vi "ImageLoader.vi"(0 "Filename":path, 1 "Load Image":bool) -> (3 "Frame 1":sgl[][](graph))   [LabVIEW 2014]
uses:
  ATSIFIO64.llb/ATSIF_ReadMode Enum.ctl
  ATSIFIO64.llb/ATSIF_DataSource Enum.ctl
panel:
  in  "stop":bool
  out "Sub Image Size":u32
  out "Sub Image Height":u32
  out "Sub Image Width":u32
  out "Image Data":sgl[](array[numeric])
  out "SubImageInfo":T1
  out "Frame Size":u32
  out "Number ofSub Images":u32
  out "Number of Frames":u32
  out "Source Present":i32
  in  "ATSIF_DataSource":T2
  out "Loaded":i32
  in  "ATSIF_ReadMode":T3
  in  "SIFPropertyValue":string
  out "SIF Property - Formatted Time":string
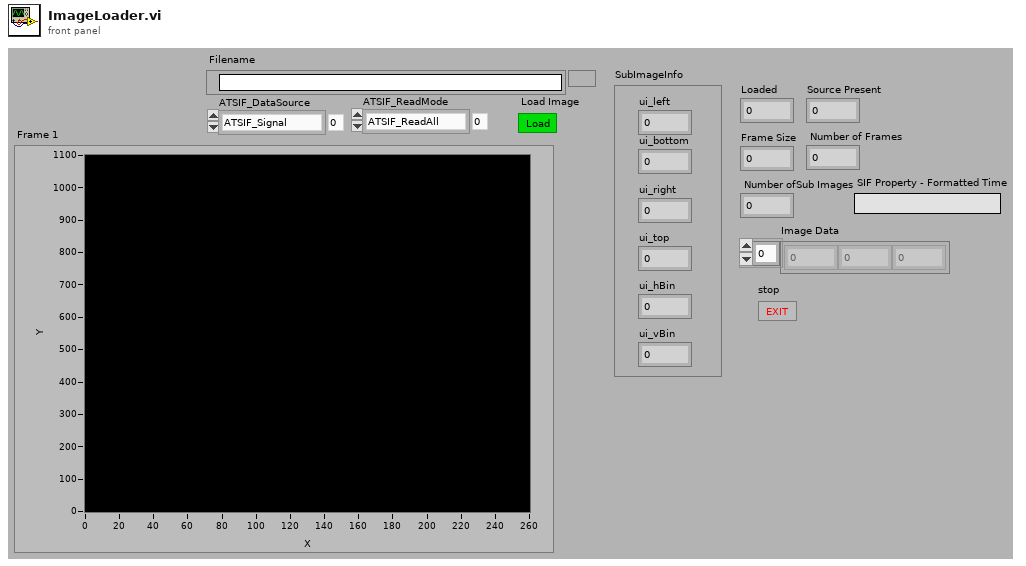
[diagram p1: front panel]
types:
  T1 = cluster{"ui_left":u32, "ui_bottom":u32, "ui_right":u32, "ui_top":u32, "ui_hBin":u32, "ui_vBin":u32}
  T2 = typedef "ATSIF_DataSource Enum.ctl" = enum16{"ATSIF_Signal", "ATSIF_Reference", "ATSIF_Background", "ATSIF_Live", "ATSIF_Source"}
  T3 = typedef "ATSIF_ReadMode Enum.ctl" = enum16{"ATSIF_ReadAll", "ATSIF_ReadHeaderOnly"}
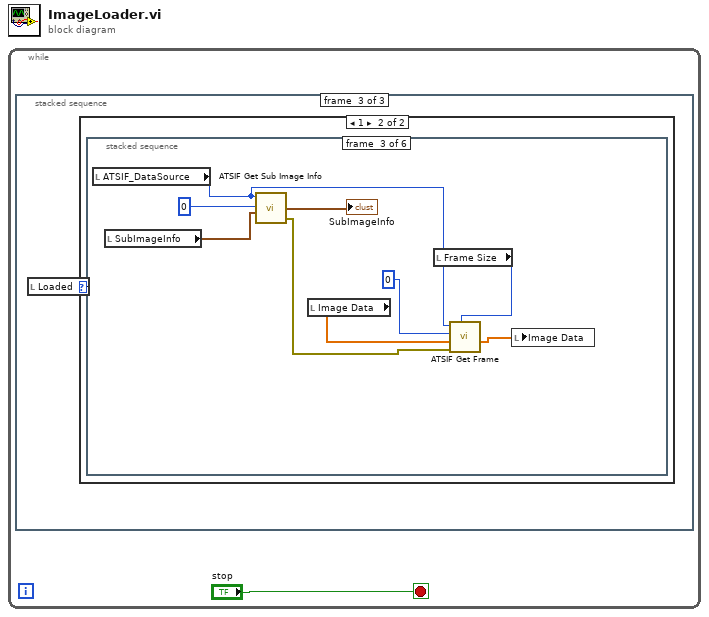
[diagram p0: block diagram]
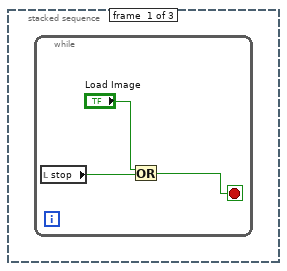
[diagram p2: hidden frame]
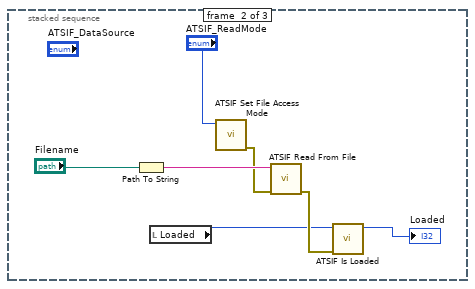
[diagram p3: hidden frame]
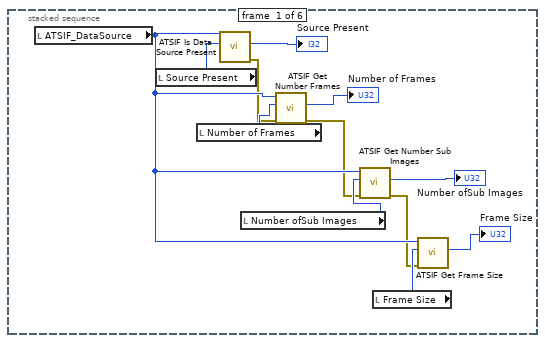
[diagram p5: hidden frame]
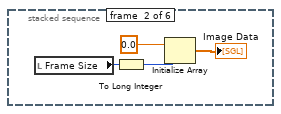
[diagram p6: hidden frame]
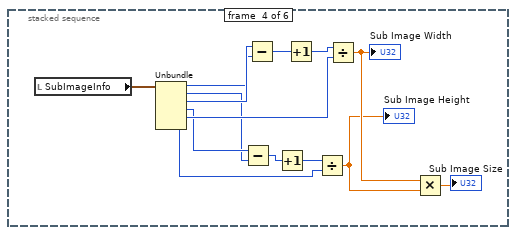
[diagram p7: hidden frame]
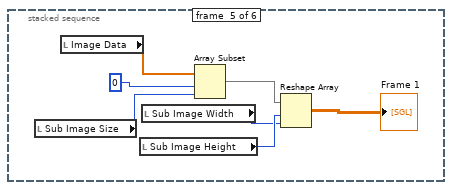
[diagram p8: hidden frame]
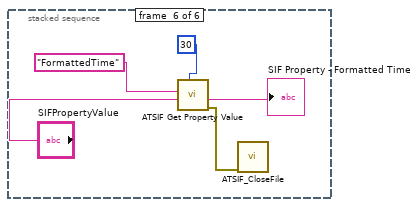
[diagram p9: hidden frame]
diagram:
  n1 = while {
    stop <- "stop" stop-if-true
    n2 = stacked-sequence {
      frame #0 {
        n3 = while {
          stop <- w3 stop-if-true
          n4 = local read "stop"() -> (w2:bool)
          n5 = Or(x="Load Image", y=w2) -> (x .or. y?=w3:bool)
        }
      }
      frame #1 {
        n6 = Path To String(path="Filename") -> (string=w11:string)
        n7 = local read "Loaded"() -> (w5:i32)
        n8 = call "ATSIF Set File Access Mode.vi"("_mode"="ATSIF_ReadMode") -> ("error out"=w7:errorcluster)  [unwired: 1 in, 9 out]
        n9 = call "ATSIF Read From File.vi"("error in (no error)"=w7, "_sz_filename"=w11) -> ("error out"=w9:errorcluster)  [unwired: 9 out]
        n10 = call "ATSIF Is Loaded.vi"("error in (no error)"=w9, "_i_loaded"=w5) -> ("_i_loaded out"=→"Loaded":i32)  [unwired: 9 out]
      }
      frame #2 {
        n11 = local read "Loaded"() -> (w12:i32)
        n12 = case shown="1" w12 {
          frame 0, Default {
          }
          frame 1 {
            n13 = stacked-sequence {
              frame #0 {
                n14 = local read "ATSIF_DataSource"() -> (w21:T2)
                n15 = local read "Source Present"() -> (w20:i32)
                n16 = local read "Number of Frames"() -> (w22:u32)
                n17 = call "ATSIF Is Data Source Present.vi"("_i_present"=w20, "_source"=w21) -> ("error out"=w18:errorcluster, "_i_present out"=→"Source Present":i32)  [unwired: 1 in, 7 out]
                n18 = local read "Number ofSub Images"() -> (w23:u32)
                n19 = call "ATSIF Get Number Frames.vi"("error in (no error)"=w18, "_ui_images"=w22, "_source"=w21) -> ("error out"=w16:errorcluster, "_ui_images out"=→"Number of Frames":u32)  [unwired: 7 out]
                n20 = call "ATSIF Get Number Sub Images.vi"("error in (no error)"=w16, "_ui_subimages"=w23, "_source"=w21) -> ("error out"=w14:errorcluster, "_ui_subimages out"=→"Number ofSub Images":u32)  [unwired: 7 out]
                n21 = local read "Frame Size"() -> (w24:u32)
                n22 = call "ATSIF Get Frame Size.vi"("error in (no error)"=w14, "_ui_size"=w24, "_source"=w21) -> ("_ui_size out"=→"Frame Size":u32)  [unwired: 8 out]
              }
              frame #1 {
                n23 = local read "Frame Size"() -> (w27:u32)
                n24 = To Long Integer(number=w27) -> (32bit integer=w26:i32)
                n25 = Initialize Array(sgl 0.0, w26) -> (→"Image Data":sgl[])
              }
              frame #2 {
                n26 = local read "ATSIF_DataSource"() -> (w32:T2)
                n27 = local read "SubImageInfo"() -> (w35:T1)
                n28 = call "ATSIF Get Sub Image Info.vi"("SubImageInfo"=w35, "_ui_index"=0, "_source"=w32) -> ("error out"=w33:errorcluster, "SubImageInfo out"=→"SubImageInfo":T1)  [unwired: 1 in, 1 out]
                n29 = local read "Image Data"() -> (w29:sgl[])
                n30 = local read "Frame Size"() -> (w31:u32)
                n31 = call "ATSIF Get Frame.vi"("_ui_bufferSize"=w31, "error in (no error)"=w33, "_pf_data"=w29, "_ui_index"=u32 0, "_source"=w32) -> ("_pf_data out"=w30:sgl[])  [unwired: 6 out]
                n32 = local write "Image Data"(w30) -> ()
              }
              frame #3 {
                n33 = local read "SubImageInfo"() -> (w51:T1)
                n34 = Unbundle(w51) -> ("ui_left"=w49:u32, "ui_bottom"=w44:u32, "ui_right"=w50:u32, "ui_top"=w45:u32, "ui_hBin"=w46:u32, "ui_vBin"=w41:u32)
                n35 = Subtract(x=w45, y=w44) -> (x-y=w43:u32)
                n36 = Subtract(x=w50, y=w49) -> (x-y=w48:u32)
                n37 = Increment(x=w43) -> (x+1=w42:u32)
                n38 = Increment(x=w48) -> (x+1=w47:u32)
                n39 = Divide(x=w42, y=w41) -> (x/y=w38:dbl)
                "Sub Image Height" <- w38
                n40 = Divide(x=w47, y=w46) -> (x/y=w39:dbl)
                "Sub Image Width" <- w39
                n41 = Multiply(x=w39, y=w38) -> (x*y=→"Sub Image Size":dbl)
              }
              frame #4 {
                n42 = local read "Sub Image Size"() -> (w56:u32)
                n43 = local read "Image Data"() -> (w58:sgl[])
                n44 = local read "Sub Image Height"() -> (w54:u32)
                n45 = local read "Sub Image Width"() -> (w53:u32)
                n46 = Array Subset(array=w58, index=0, length=w56) -> (w55:sgl[])
                n47 = Reshape Array(w55, w54, w53) -> (→"Frame 1":sgl[][])
              }
              frame #5 {
                n48 = call "ATSIF Get Property Value.vi"("_sz_propertyName"="FormattedTime", "_sz_propertyValue"="SIFPropertyValue", "_ui_bufferSize"=u32 30) -> ("_sz_propertyValue out"=→"SIF Property - Formatted Time":string, "error out"=w59:errorcluster)  [unwired: 2 in, 4 out]
                n49 = call "ATSIF_CloseFile.vi"("error in (no error)"=w59) -> ()  [unwired: 11 out]
              }
            }
          }
        }
      }
    }
  }
